vi "Run Service.vi"() -> ()   [LabVIEW 2020, in "Veristandgrpc_server.lvlib"]
uses:
  Veristandgrpc_server.lvlib
  <vilib>/gRPC/LabVIEW gRPC Servicer/Servicer/Servicer.lvclass/Servicer.ctl
  RPC Service/veristand/veristand-grpc.lvclass
  C:/Program Files (x86)/National Instruments/LabVIEW 2020/vi.lib/gRPC/LabVIEW gRPC Servicer/ServiceBase/ServiceBase.lvclass
  Data/Data Server.lvclass/Data Server.ctl
  Data/Data Server.lvclass
  <vilib>/gRPC/LabVIEW gRPC Servicer/Servicer/Servicer.lvclass
  <vilib>/gRPC/LabVIEW gRPC Servicer/ServiceBase/ServiceBase.lvclass
panel:
  in  "Data in Memory":string[][](table)=[["Test", "Dummy"], ["Operator", "John"], ["DUT", "Golden"], ["Serial Number", "0xAB"], ["Timestamp", "5/1/2023"]]
  in  "Async [T] / Sync [F]":bool
  out "Listening Port":i32
  in  "Stop":bool
  in  "Server Address":string="localhost:50051"
  in  "Server Certificate File (.crt)":path
  in  "Server Key File (.key)":path
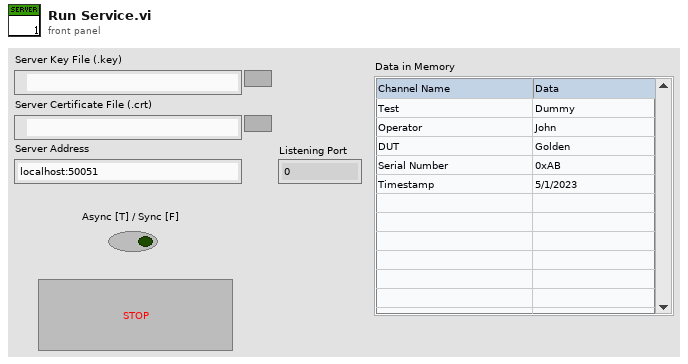
[diagram p1: front panel]
types:
  T1 = typedef "grpc-lvsupport-release.lvlib/grpcId.ctl" = u64
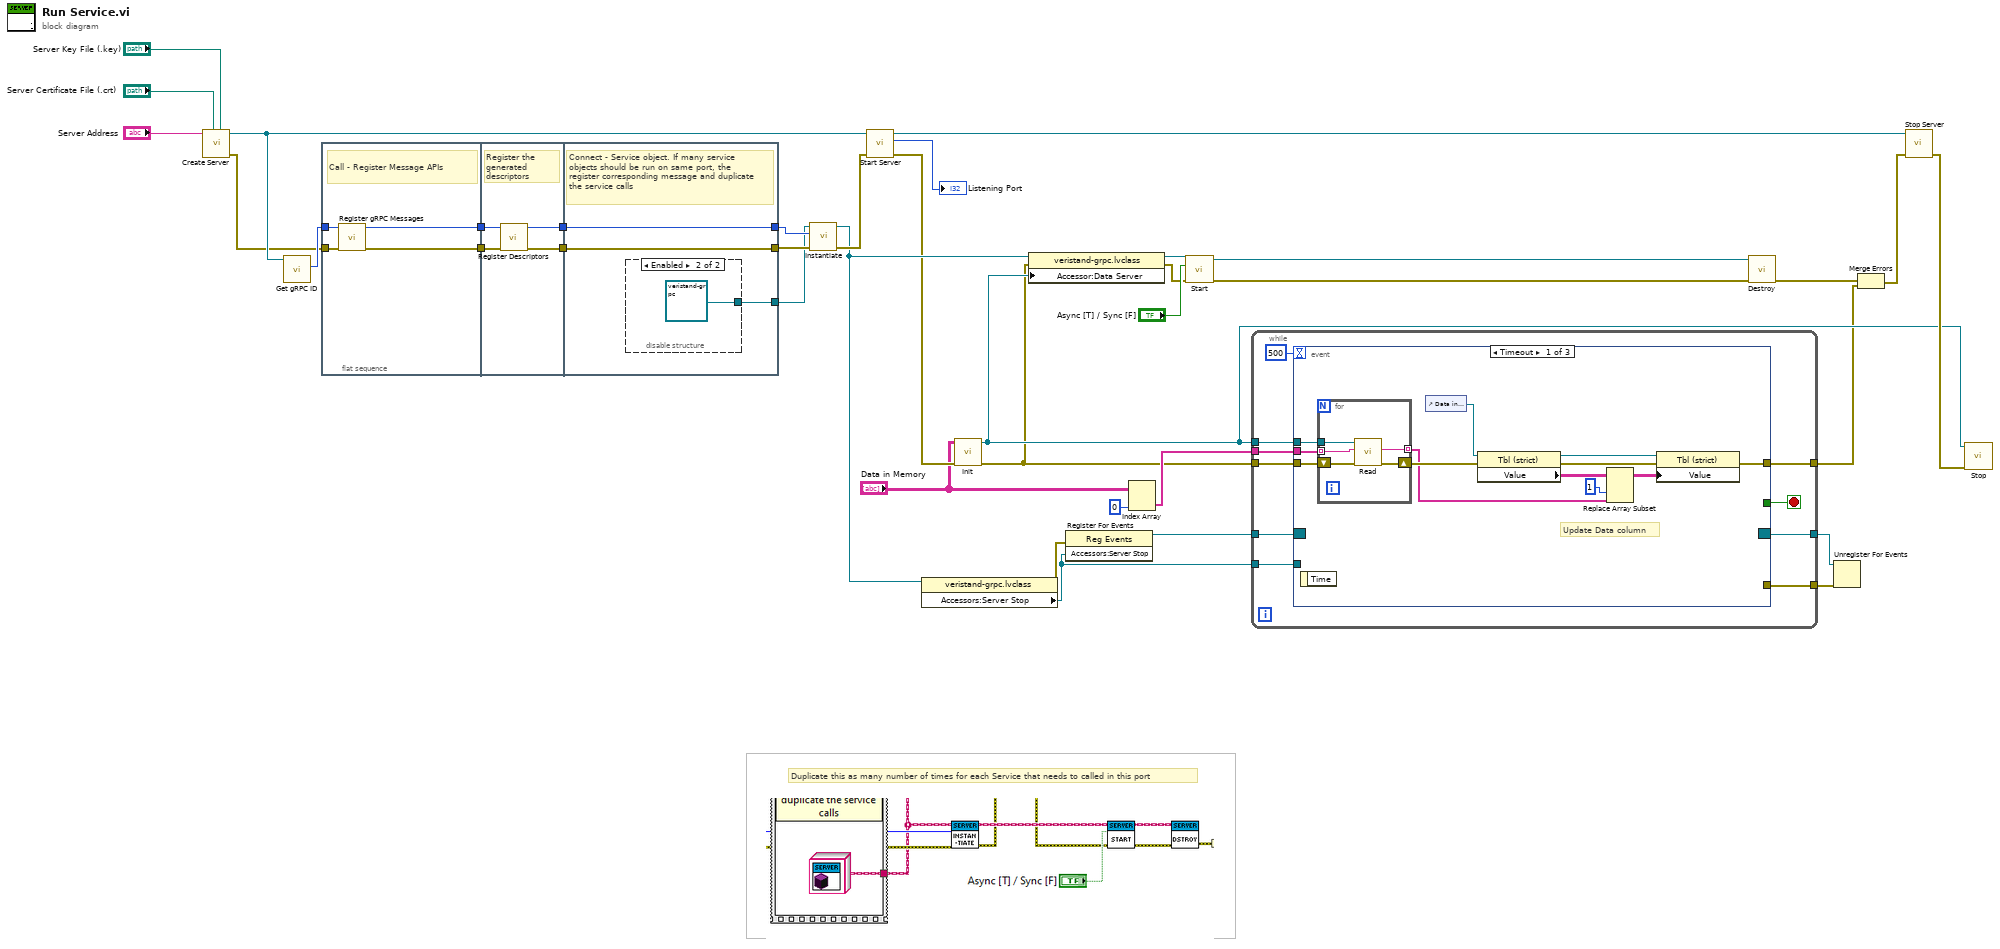
[diagram p0: block diagram]
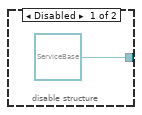
[diagram p2: hidden frame]
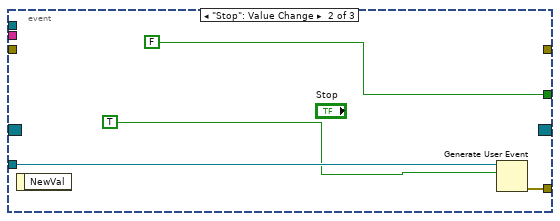
[diagram p3: hidden frame]
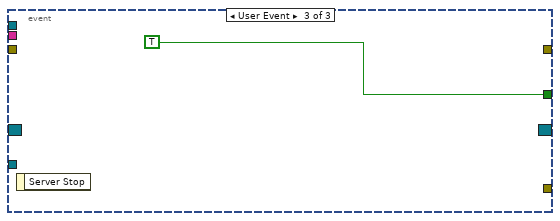
[diagram p4: hidden frame]
diagram:
  # "Duplicate this as many number of times for each Service that needs to called in this port"
  n1 = call <vilib>:"Create Server.vi"("Server Key File (.key)"="Server Key File (.key)", "Server Certificate File (.crt)"="Server Certificate File (.crt)", "Server Address"="Server Address") -> ("error out"=w23:errorcluster, "gRPC Server out"=w30:refnum<class "Servicer.lvclass">)  [unwired: 7 in]
  n2 = call <vilib>:"Get gRPC ID.vi"("OOP Server in"=w30) -> ("gRPC ID"=w24:T1)  [unwired: 9 in, 1 out]
  n3 = flat-sequence {
    tunnel: w24 -> [w39]
    tunnel: w23 -> [w41]
    tunnel: [w40] -> w17
    tunnel: [w38] -> w16
    tunnel: w17 -> [w44]
    tunnel: w16 -> [w45]
    tunnel: [w42] -> w15
    tunnel: [w43] -> w14
    tunnel: [w47] -> w21
    tunnel: [w48] -> w22
    tunnel: w15 -> [w48]
    tunnel: w14 -> [w47]
    tunnel: [w46] -> w13
    frame #0 {
      # "Call - Register Message APIs"
      n4 = call "Register gRPC Messages.vi"("error in (no error)"=w41, "gRPC ID"=w39) -> ("error out"=w40:errorcluster, "gRPC ID Out"=w38:T1)  [unwired: 8 in]
    }
    frame #1 {
      # "Register the generated descriptors"
      n5 = call "Register Descriptors.vi"("error in (no error)"=w44, "gRPC ID"=w45) -> ("error out"=w42:errorcluster, "gRPC ID Out"=w43:T1)  [unwired: 8 in]
    }
    frame #2 {
      # "Connect - Service object. If many service objects should be run on same port, the register corresponding message and duplicate the service calls"
      n6 = disable-structure shown="Enabled" {
        disable-tunnel: [refnum<class "ServiceBase.lvclass"> refnum ("gRPC-servicer.lvlib:iService.lvclass") refnum<class "veristand-grpc.lvclass"> refnum ("veristand-grpc_server.lvlib:veristand.lvclass")] -> w46
        frame Disabled {
        }
        frame Enabled {
        }
      }
    }
  }
  n7 = call-dynamic "Instantiate.vi"("error in"=w22, "gRPCid"=w21, "iService"=w13) -> ("error out"=w28:errorcluster, "iService"=w12:refnum<class "veristand-grpc.lvclass">)  [unwired: 7 in]
  n8 = call <vilib>:"Start Server.vi"("error in"=w28, "gRPC Server in"=w30) -> ("error out"=w9:errorcluster, "Listening Port"=→"Listening Port":i32, "gRPC Server out"=w37:refnum<class "Servicer.lvclass">)  [unwired: 7 in]
  n9 = property class="veristand-grpc.lvclass"(reference=w12) -> (error out=w29:errorcluster, "Accessors:Server Stop"=w18:refnum<user-event>)  [unwired: 1 in, 1 out]
  n10 = call "Init.vi"("error in (no error)"=w9, "Initial Data"="Data in Memory") -> ("error out"=w2:errorcluster, "DVR out"=w6:refnum<class "Data Server.lvclass">)  [unwired: 8 in]
  n11 = property class="veristand-grpc.lvclass"(reference=w12, error in=w2, "Accessor:Data Server"=w6) -> (reference out=w11:refnum<class "veristand-grpc.lvclass">, error out=w10:errorcluster)
  n12 = register-events(error in=w29, w18) -> (reference out=w33:refnum<event-registration>)  [unwired: 1 in, 1 out]
  n13 = Index Array(array="Data in Memory", index (col)=0 ("disabled index (col)")) -> (element=w3:string[])  [unwired: 1 in]
  n14 = call-dynamic "Start.vi"("error in"=w10, "ASync [T]"="Async [T] / Sync [F]", "iService in"=w11) -> ("error out"=w8:errorcluster, "iService out"=w20:refnum<class "veristand-grpc.lvclass">)  [unwired: 7 in]
  n15 = while {
    tunnel: w33 -> [w60]
    tunnel: [w58] -> w32
    tunnel: [w56] -> w25
    tunnel: w18 -> [w57]
    tunnel: w6 -> [w54]
    tunnel: w2 -> [w53]
    tunnel: [w52] -> w5
    tunnel: w3 -> [w51]
    stop <- w59 stop-if-true
    n16 = event shown="[0] Timeout" {
      selector: w60 -> [_ _ _]
      dyn-events: [_ _ _] -> w58
      timeout: 500 -> [_ _ _]
      tunnel: [_ FALSE TRUE] -> w59
      tunnel: w57 -> [_ w80 _]
      tunnel: [_ w78 _] -> w56
      tunnel: w54 -> [w72 _ _]
      tunnel: w53 -> [w71 _ _]
      tunnel: [w62 _ _] -> w52
      tunnel: w51 -> [w64 _ _]
      event Timeout {
        # "Update Data column"
        n17 = event-data() -> ()  [unwired: 1 in, 1 out]
        n18 = for {
          tunnel: w72 -> [w77]
          shift-right: [w75] -> w63
          shift-left: w71 -> [w76]
          tunnel: w64 -> [w74] mode=indexing
          tunnel: [w73] -> w61 mode=indexing
          n19 = call "Read.vi"("error in (no error)"=w76, "Channel Name"=w74, "Data in"=w77) -> ("error out"=w75:errorcluster, "Data"=w73:string)  [unwired: 5 in, 2 out]
        }
        n20 = control-ref of="Data in Memory"() -> (w65:refnum<vi>)
        n21 = property class="Tbl (strict)"(reference=w65, error in=w63) -> (reference out=w68:refnum<vi>, error out=w67:errorcluster, "Value"=w70:string[][])
        n22 = Replace Array Subset(array=w70, new element=w61, index (col)=1 ("disabled index (col)")) -> (w69:string[][])  [unwired: 1 in]
        n23 = property class="Tbl (strict)"(reference=w68, error in=w67, "Value"=w69) -> (error out=w62:errorcluster)  [unwired: 1 out]
      }
      event "Stop": Value Change {
        n24 = event-data() -> ()  [unwired: 1 in, 1 out]
        n25 = Generate User Event(user event=w80, event data cluster=TRUE ("event data")) -> (error out=w78:errorcluster)  [unwired: 2 in, 1 out]
      }
      event User Event {
        n26 = event-data() -> ()  [unwired: 1 in, 1 out]
      }
    }
  }
  n27 = call-dynamic "Destroy.vi"("error in (no error)"=w8, "SignalGeneratorService in"=w20) -> ("error out"=w27:errorcluster)  [unwired: 8 in, 1 out]
  n28 = Unregister For Events(event registration refnum=w32, error in=w25) -> ()  [unwired: 1 out]
  n29 = Merge Errors(w27, w5) -> (w26:errorcluster)
  n30 = call <vilib>:"Stop Server.vi"("error in"=w26, "gRPC Server in"=w37) -> ("error out"=w7:errorcluster)  [unwired: 9 in]
  n31 = call "Stop.vi"("error in (no error)"=w7, "DVR in"=w6) -> ()  [unwired: 9 in, 1 out]
